vi "FTW-JSON-GetElementInfo.vi"(0 "JSON":T2, 5 "Path to Element":string, 11 "error in":errorcluster) -> (4 "JSON out":T2, 6 "Element Type":T1, 8 "Contained Elements":i32, 15 "error out":errorcluster)   [LabVIEW 2015]
uses:
  core/type/FTW-Type-JSON.ctl
  FTW-JSON-Type.ctl
  core/FTW-JSON-Core-Type.ctl
panel:
  # "Inputs"
  # "Outputs"
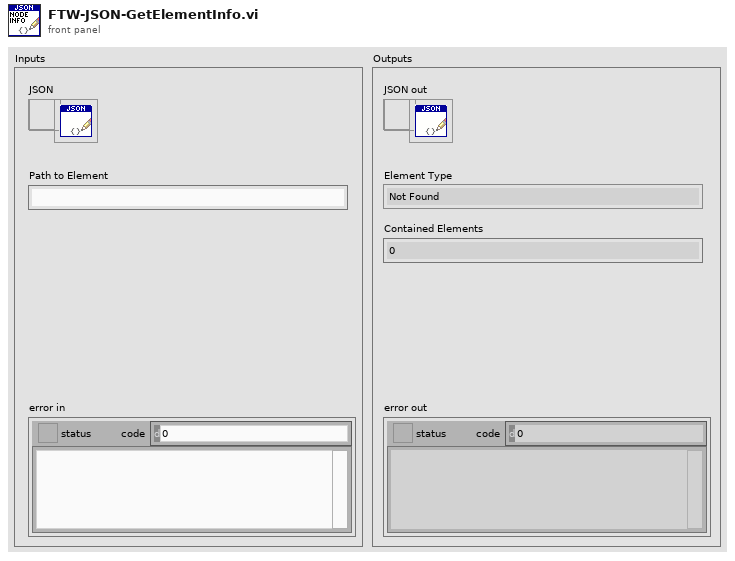
[diagram p1: front panel]
types:
  T1 = typedef "FTW-JSON-Type.ctl" = enum8{"Not Found", "Object", "Array", "String", "Number", "Boolean", "null"}
  T2 = typedef "FTW-Type-JSON.ctl" = refnum<data-value>
  T3 = typedef "FTW-JSON-Core-Type.ctl" = enum8{"Object", "Array", "String", "Integer", "Floating Point", "true", "false", "null", "undefined"}
  T4 = cluster{"FTW-CodeGen-Type":enum16{"FTW-JSON"}, "Object":i64, "EncodingFlags":i64, "DecodingFlags":i64}
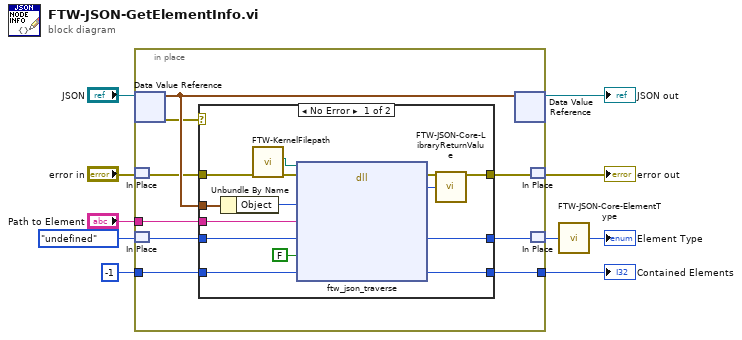
[diagram p0: block diagram]
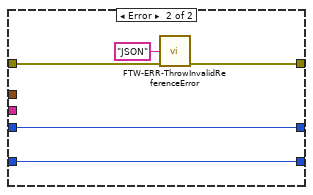
[diagram p2: hidden frame]
diagram:
  n1 = in-place {
    in-place-border: "Path to Element" -> [w17]
    in-place-border: [w12] -> w2
    in-place-border: -1 -> [w11]
    n2 = in-place-dvr #1("JSON") -> (w19:T4, w18:errorcluster)
    n3 = in-place-match #2("error in") -> (w16:errorcluster)
    n4 = in-place-match #3(FTW-JSON-Core-Type."undefined" ("Actual Type")) -> (w14:T3)
    n5 = case shown="No Error" w18 {
      tunnel: w16 -> [w32 w38]
      tunnel: [w25 w37] -> w15
      tunnel: w19 -> [w33 _]
      tunnel: w17 -> [w28 _]
      tunnel: w14 -> [w27 w35]
      tunnel: [w22 w35] -> w13
      tunnel: [w21 w34] -> w12
      tunnel: w11 -> [w20 w34]
      frame No Error {
        n6 = Unbundle By Name(w33) -> ("Object"=w29:i64)
        n7 = call "FTW-KernelFilepath.vi"("error in"=w32) -> ("error out"=w30:errorcluster, "Library Filepath"=w31:path)  [unwired: 8 in, 1 out]
        n8 = dll-call lib="?" fn="ftw_json_traverse"(path in=w31, error in=w30, "JSON Element"=w29, "JSON Path"=w28, "Actual Type"=w27, "Remove"=FALSE, "Num Elements"=w20) -> (error out=w26:errorcluster, "Return Code"=w23:i64, "Actual Type"=w22:T3, "Num Elements"=w21:i32)  [unwired: 4 in, 1 out]
        n9 = call "FTW-JSON-Core-LibraryReturnValue.vi"("error in"=w26, "Return Code"=w23) -> ("error out"=w25:errorcluster)  [unwired: 13 in]
      }
      frame Error {
        n10 = call "FTW-ERR-ThrowInvalidReferenceError.vi"("Reference Type"="JSON", "error in"=w38) -> ("error out"=w37:errorcluster)  [unwired: 13 in]
      }
    }
    n11 = in-place-dvr #1(w19) -> (→"JSON out":T2)  [unwired: 1 out]
    n12 = in-place-match #2(w15) -> (→"error out":errorcluster)
    n13 = in-place-match #3(w13) -> (w4:T3)
  }
  "Contained Elements" <- w2
  n14 = call "FTW-JSON-Core-ElementType.vi"("Core Type"=w4) -> ("JSON Element Type"=→"Element Type":T1)
